vi "Create Folder.vi"(8 "error in (no error)":errorcluster, 10 "Name":string, 11 "Path in":path) -> (0 "error out":errorcluster, 2 "Original Path":path, 3 "new Path":path)   [LabVIEW 2019]
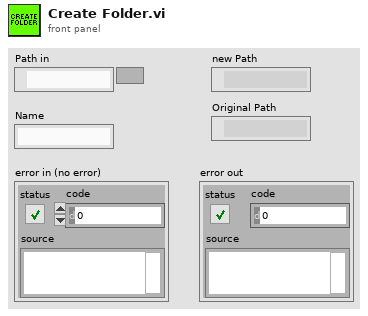
[diagram p1: front panel]
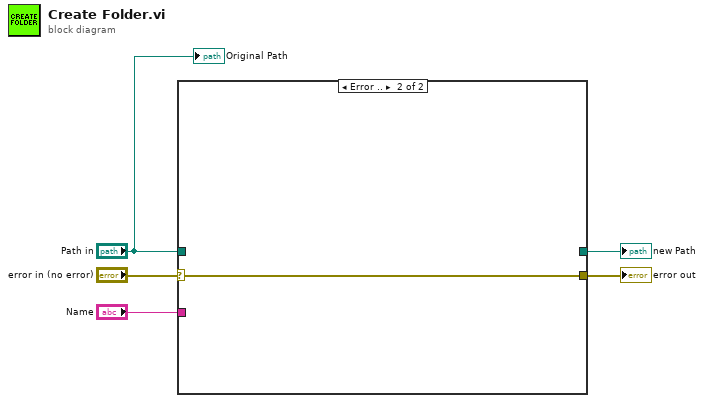
[diagram p0: block diagram]
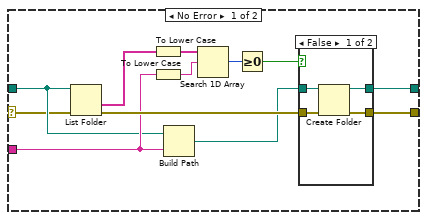
[diagram p2: hidden frame]
diagram:
  n1 = case shown="Error .." "error in (no error)" {
    selector: "error in (no error)" -> [w6 w23]
    tunnel: [w17 w23] -> w5
    tunnel: [w15 _] -> w4
    tunnel: "Name" -> [w14 _]
    tunnel: "Path in" -> [w7 _]
    frame No Error {
      n2 = List Folder(path=w7, error in=w6) -> (folder names=w13:string[], error out=w16:errorcluster)  [unwired: 2 in, 2 out]
      n3 = To Lower Case(string=w13) -> (all lower case string=w8:string[])
      n4 = To Lower Case(string=w14) -> (all lower case string=w9:string)
      n5 = Build Path(base path=w7, name or relative path=w14) -> (appended path=w12:path)
      n6 = Search 1D Array(1D array=w8, element=w9) -> (index of element=w10:i32)  [unwired: 1 in]
      n7 = Greater Or Equal To 0?(x=w10) -> (x >= 0?=w11:bool)
      n8 = case shown="False" w11 {
        tunnel: w12 -> [w21 w22]
        tunnel: [w20 w22] -> w15
        tunnel: [w19 _] -> w17
        tunnel: w16 -> [w18 _]
        frame False {
          n9 = Create Folder(path (use dialog)=w21, error in=w18) -> (created path=w20:path, error out=w19:errorcluster)  [unwired: 1 in, 1 out]
        }
        frame True {
        }
      }
    }
    frame Error {
    }
  }
  "error out" <- w5
  "new Path" <- w4
  "Original Path" <- "Path in"
